vi "FlipfFlopT.vi"(10 "Q":bool, 11 "T":bool) -> (2 "Q\\*":bool, 3 "Q*":bool)   [LabVIEW 2018]
panel:
  out "Title":string="FlipFlopT"
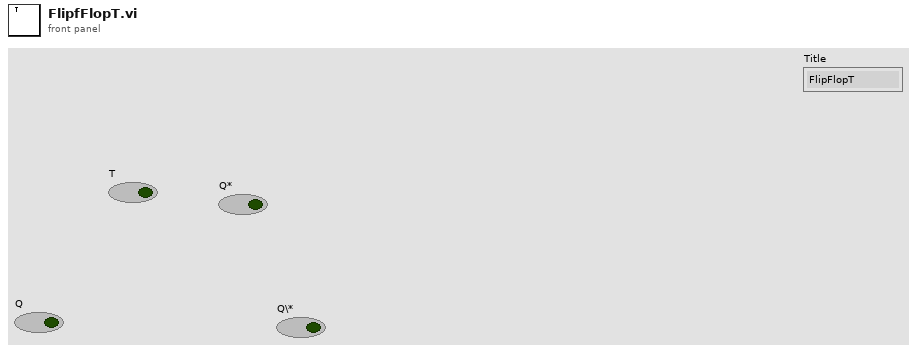
[diagram p1: front panel]
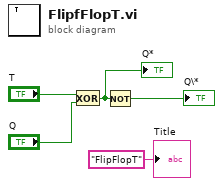
[diagram p0: block diagram]
diagram:
  n1 = Exclusive Or(1:"Q", 2:"T") -> (0:w4:bool)
  "Q*" <- w4
  n2 = Not(x=w4) -> (.not. x?=→"Q\\*":bool)
  "Title" <- "FlipFlopT"
